vi "PCAN_CompLaserPosition.vi"(1 "Laser 4":dbl, 2 "Laser 3":dbl, 3 "Laser 2":dbl, 4 "Laser 1":dbl) -> (0 "Array":u8[](array[numeric]))   [LabVIEW 2013]
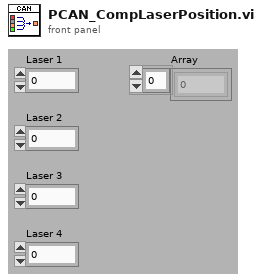
[diagram p1: front panel]
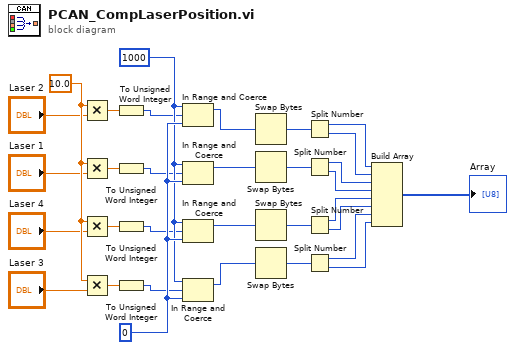
[diagram p0: block diagram]
diagram:
  w13 = 10.0 ("x")
  w15 = u16 0 ("lower limit")
  w14 = u16 1000 ("upper limit")
  n1 = Multiply(x=w13, y="Laser 2") -> (x*y=w9:dbl)
  n2 = Multiply(x=w13, y="Laser 1") -> (x*y=w10:dbl)
  n3 = Multiply(x=w13, y="Laser 4") -> (x*y=w11:dbl)
  n4 = Multiply(x=w13, y="Laser 3") -> (x*y=w12:dbl)
  n5 = To Unsigned Word Integer(number=w9) -> (unsigned 16bit integer=w8:u16)
  n6 = To Unsigned Word Integer(number=w10) -> (unsigned 16bit integer=w7:u16)
  n7 = To Unsigned Word Integer(number=w11) -> (unsigned 16bit integer=w6:u16)
  n8 = To Unsigned Word Integer(number=w12) -> (unsigned 16bit integer=w5:u16)
  n9 = In Range and Coerce(upper limit=w14, x=w8, lower limit=w15) -> (coerced(x)=w19:u16)  [unwired: 1 out]
  n10 = In Range and Coerce(upper limit=w14, x=w7, lower limit=w15) -> (coerced(x)=w16:u16)  [unwired: 1 out]
  n11 = In Range and Coerce(upper limit=w14, x=w6, lower limit=w15) -> (coerced(x)=w17:u16)  [unwired: 1 out]
  n12 = In Range and Coerce(upper limit=w14, x=w5, lower limit=w15) -> (coerced(x)=w18:u16)  [unwired: 1 out]
  n13 = Swap Bytes(anything=w19) -> (byte swapped=w21:u16)
  n14 = Swap Bytes(anything=w16) -> (byte swapped=w22:u16)
  n15 = Swap Bytes(anything=w17) -> (byte swapped=w27:u16)
  n16 = Swap Bytes(anything=w18) -> (byte swapped=w28:u16)
  n17 = Split Number(x=w21) -> (hi(x)=w23:u8, lo(x)=w24:u8)
  n18 = Split Number(x=w22) -> (hi(x)=w25:u8, lo(x)=w26:u8)
  n19 = Split Number(x=w27) -> (hi(x)=w29:u8, lo(x)=w32:u8)
  n20 = Split Number(x=w28) -> (hi(x)=w31:u8, lo(x)=w30:u8)
  n21 = Build Array(w23, w24, w25, w26, w29, w32, w31, w30) -> (→"Array":u8[])
